vi "Write Value.vi"(8 "error in (no error)":errorcluster, 10 "Abs_Numeric.lvclass":refnum<class "Abs_Numeric.lvclass">, 11 "ConvertTo_DBL in":refnum<class "ConvertTo_U16.lvclass">) -> (0 "error out":errorcluster, 3 "ConvertTo_DBL out":refnum<class "ConvertTo_U16.lvclass">)   [LabVIEW 2021, in "ConvertTo_U16.lvclass"]
uses:
  ConvertTo_U16.lvclass
  Abs_Types/Numeric/Abs_Numeric.lvclass
  ConvertTo_U16.lvclass/ConvertTo_U16.ctl
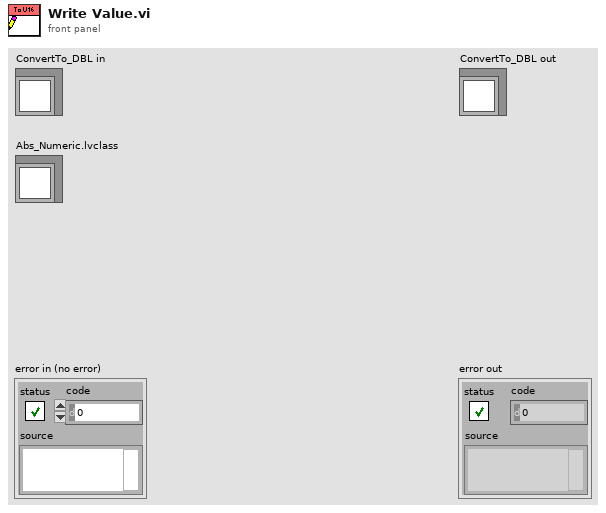
[diagram p1: front panel]
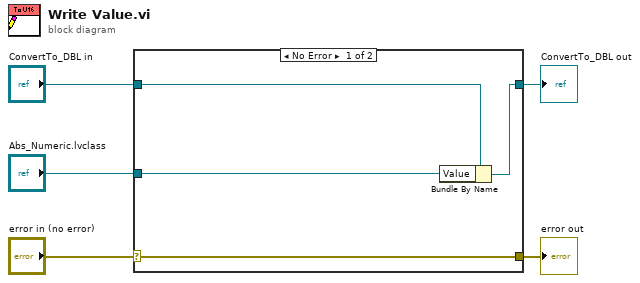
[diagram p0: block diagram]
diagram:
  n1 = case shown="No Error" "error in (no error)" {
    selector: "error in (no error)" -> [w9 w10]
    tunnel: [w9 w10] -> w4
    tunnel: [w7 w11] -> w2
    tunnel: "ConvertTo_DBL in" -> [w8 w11]
    tunnel: "Abs_Numeric.lvclass" -> [w6 _]
    frame No Error {
      n2 = Bundle By Name(cluster=w8, "Value"=w6) -> (w7:refnum<class "ConvertTo_U16.lvclass">)
    }
    frame Error {
    }
  }
  "error out" <- w4
  "ConvertTo_DBL out" <- w2
